vi "Read Results from processing.vi"(8 "error in":errorcluster, 11 "DAQmx Watchdog runtime in":refnum<class "DAQmx Watchdog runtime.lvclass">) -> (0 "error out":errorcluster, 2 "Results from processing":T1, 3 "DAQmx Watchdog runtime out":refnum<class "DAQmx Watchdog runtime.lvclass">)   [LabVIEW 2014]
uses:
  DAQmx Watchdog runtime.lvclass
  configuration/result data indices.ctl
  configuration/DAQmx Watchdog configuration.lvclass
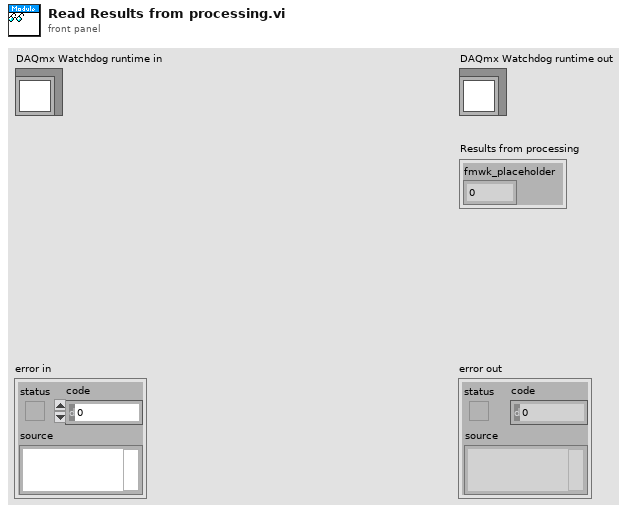
[diagram p1: front panel]
types:
  T1 = typedef "DAQmx Watchdog configuration.lvclass/result data indices.ctl" = cluster{"fmwk_placeholder":i32}
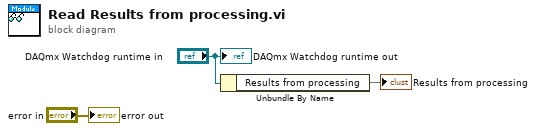
[diagram p0: block diagram]
diagram:
  n1 = Unbundle By Name("DAQmx Watchdog runtime in") -> ("Results from processing"=→"Results from processing")
  "error out" <- "error in"
  "DAQmx Watchdog runtime out" <- "DAQmx Watchdog runtime in"
